vi "rqcBob Modulator Config.vi"(0 "rqcBob in":refnum<class "rqcBob.lvclass">, 5 "Modulator.Start":u16, 7 "Modulator.Stop":u16, 9 "Modulator.Clock Delay":fxp<+,4,4>, 11 "error in (no error)":errorcluster, 12 "Modulator.Value Type":T1=enum."constant", 13 "DAC value":u16=150) -> (4 "rqcBob out":refnum<class "rqcBob.lvclass">, 15 "error out":errorcluster)   [LabVIEW 2019, in "rqcBob.lvclass"]
uses:
  rqcBob.lvclass
  Shared/Shared FPGA Lib/Shared Logic/Custom Controls/rqc Random Generator.value type.ctl
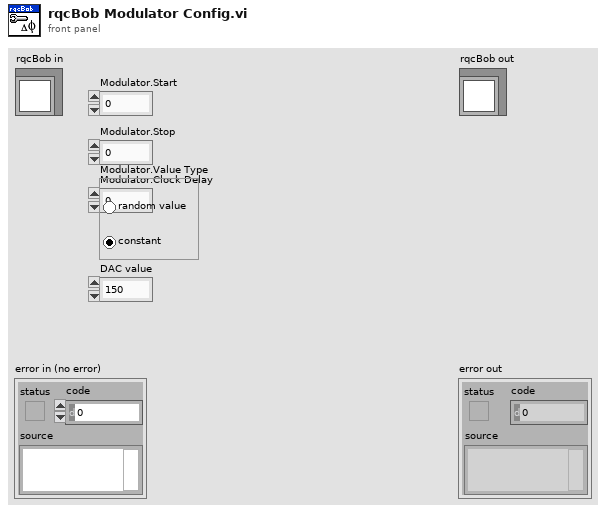
[diagram p1: front panel]
types:
  T1 = typedef "rqc Random Generator.value type.ctl" = enum32{"random value", "constant"}
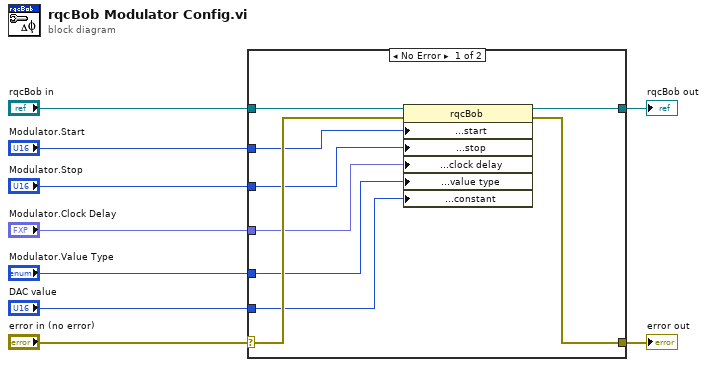
[diagram p0: block diagram]
diagram:
  n1 = case shown="No Error" "error in (no error)" {
    selector: "error in (no error)" -> [w16 w20]
    tunnel: [w15 w20] -> w8
    tunnel: [w17 w19] -> w6
    tunnel: "rqcBob in" -> [w18 w19]
    tunnel: "Modulator.Start" -> [w14 _]
    tunnel: "Modulator.Stop" -> [w13 _]
    tunnel: "Modulator.Clock Delay" -> [w12 _]
    tunnel: "Modulator.Value Type" -> [w11 _]
    tunnel: "DAC value" -> [w10 _]
    frame No Error {
      n2 = property class="rqcBob"(reference=w18, error in=w16, "public:Public Properties Access:Modulator:modulator.start"=w14, "public:Public Properties Access:Modulator:modulator.stop"=w13, "public:Public Properties Access:Modulator:modulator.clock delay"=w12, "public:Public Properties Access:Random Number Generator:value type"=w11, "public:Public Properties Access:Random Number Generator:constant"=w10) -> (reference out=w17:refnum<class "rqcBob.lvclass">, error out=w15:errorcluster)
    }
    frame Error {
    }
  }
  "error out" <- w8
  "rqcBob out" <- w6
